vi "Vision Research Phantom Series Unregister Client.vi"(5 "Error In (no error)":errorcluster) -> (14 "HRESULT":i32, 19 "Error Out":errorcluster)   [LabVIEW 2013, in "VRI.lvlib"]
doc: "PhCon.dll\n\nThis VI unregisters the client from the Vision Research Phantom Series camera using the PhCon dll.\n\nPhUnregisterClient\nHRESULT PhUnregisterClient() ;\n\nParameters Description\nReturn HRESULT (0=Ok)\nComments Ends the registration.\n\nWritten by:\nBLOOMY CONTROLS, INC\nWINDSOR, CT 06095, USA\n860-298-9925\nwww.bloomy.com\nV1.0.0\nMay, 2004"
uses:
  VRI.lvlib
  Phantom DLLs/PhCon.dll
panel:
  # "For instructions on the use of this VI, press Ctrl+H to display the help window and move the mouse over the icon, controls, and indicators"
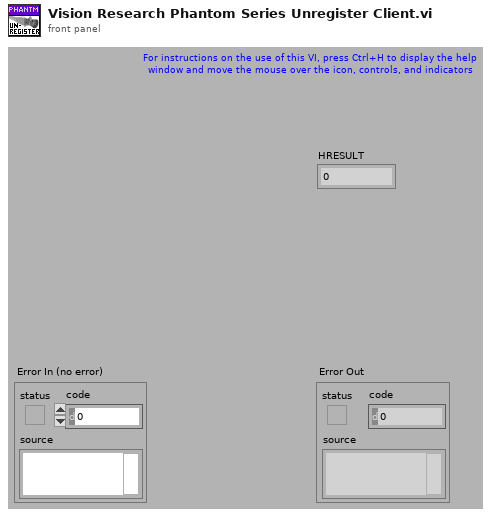
[diagram p1: front panel]
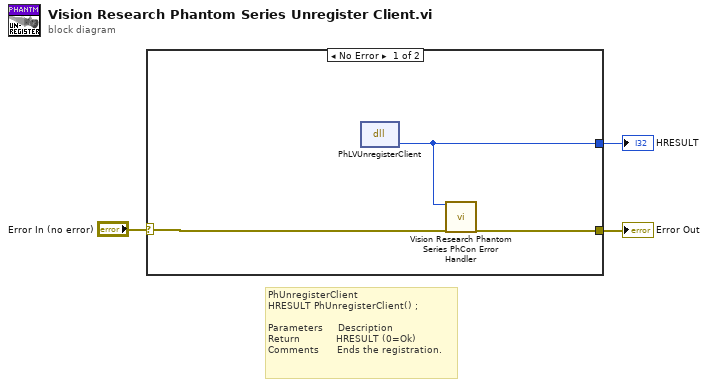
[diagram p0: block diagram]
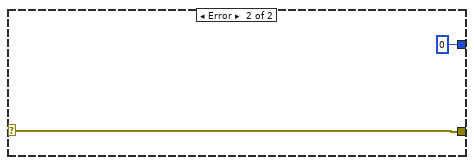
[diagram p2: hidden frame]
diagram:
  # "PhUnregisterClient\nHRESULT PhUnregisterClient() ;\n\nParameters     Description\nReturn            HRESULT (0=Ok)\nComments      Ends the registration."
  n1 = case shown="No Error" "Error In (no error)" {
    selector: "Error In (no error)" -> [w6 w8]
    tunnel: [w5 w8] -> w2
    tunnel: [w4 0] -> w1
    frame No Error {
      n2 = dll-call lib="C:/Projects/SDK/32-bit/Vision Research Phantom Series Labview Driver/Phantom DLLs/PhCon.dll" fn="PhLVUnregisterClient"() -> ("HRESULT"=w4:i32)  [unwired: 3 in, 2 out]
      n3 = call "Vision Research Phantom Series PhCon Error Handler.vi"("ErrNo"=w4, "Error In (no error)"=w6) -> ("Error Out"=w5:errorcluster)  [unwired: 17 out]
    }
    frame Error {
    }
  }
  "Error Out" <- w2
  "HRESULT" <- w1
